vi "Open sequence.vi"(7 "Sequence name":string, 11 "error in (no error)":errorcluster) -> (4 "User input 1":T1, 6 "string steps":string[](array[string]), 8 "Steps":T2[](array[typedef]), 10 "Problem reading sequence":bool, 15 "error out":errorcluster)   [LabVIEW 2011]
uses:
  Sequence steps config..ctl
  Single criteria cluster.ctl
  Criteria types.ctl
  Boolean operation.ctl
  User input.ctl
  <vilib>/Utility/config.llb/NI_LVConfig.lvlib
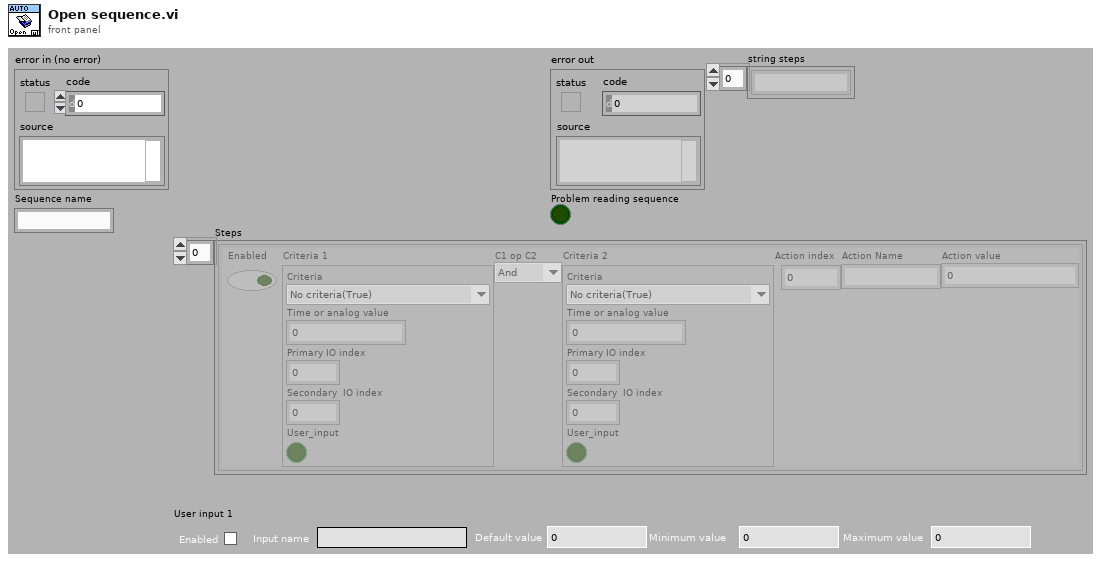
[diagram p1: front panel]
types:
  T1 = typedef "User input.ctl" = cluster{"Input name":string, "Minimum value ":dbl, "Maximum value":dbl, "Default value":dbl, "User inp enabled":bool}
  T2 = typedef "Sequence steps config..ctl" = cluster{"Enabled":bool, "Criteria 1":T3, "C1 op C2":T5, "Criteria 2":T3, "Action index":i32, "Action Name":string, "Action value":dbl}
  T3 = typedef "Single criteria cluster.ctl" = cluster{"Criteria":T4, "Time or analog value":dbl, "Primary IO index":i32, "Secondary  IO index":i32, "User_input":bool}
  T4 = typedef "Criteria types.ctl" = enum16{"No criteria(True)", "Time(s)", "Analog IO over", "Analog IO over or equal", "Analog IO under", "Analog IO under or equal", "Analog IO 1 minus Analog IO 2 over", "Digital IO True", "Digital IO False", "Operator approval"}
  T5 = typedef "Boolean operation.ctl" = enum16{"And", "Or", "Xor", "Nand", "Nor", "Nxor", "Implies"}
  T6 = typedef "NI_LVConfig.lvlib/Config Data RefNum.ctl" = refnum<k1>
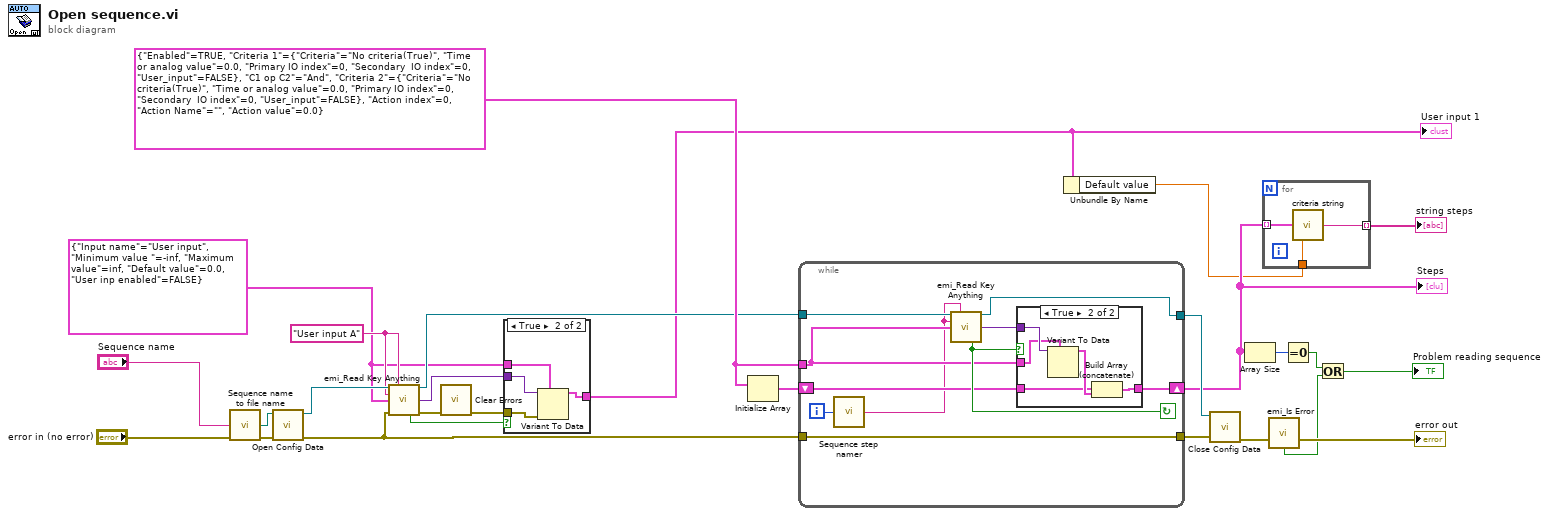
[diagram p0: block diagram]
diagram:
  w3 = T1 {"Input name"="User input", "Minimum value "=-inf, "Maximum value"=inf, "Default value"=0.0, "User inp enabled"=FALSE} ("User input 1")
  w7 = "User input A" ("Section(Default)")
  w21 = T2 {"Enabled"=TRUE, "Criteria 1"={"Criteria"=enum."No criteria(True)", "Time or analog value"=0.0, "Primary IO index"=0, "Secondary  IO index"=0, "User_input"=FALSE}, "C1 op C2"=enum."And", "Criteria 2"={"Criteria"=enum."No criteria(True)", "Time or analog value"=0.0, "Primary IO index"=0, "Secondary  IO index"=0, "User_input"=FALSE}, "Action index"=0, "Action Name"="", "Action value"=0.0} ("data step cluster")
  n1 = call "Sequence name to file name.vi"("Sequence name"="Sequence name", "error in (no error)"="error in (no error)") -> ("Sequence file path"=w25:path, "error out"=w24:errorcluster)  [unwired: 12 in]
  n2 = call <vilib>:"Open Config Data.vi"("error in (no error)"=w24, "configuration file path"=w25) -> ("error out"=w11:errorcluster, "refnum"=w9:T6)  [unwired: 7 in, 1 out]
  n3 = call "emi_Read Key Anything.vi"("Ini file refnum"=w9, "Section(Default)"=w7, "Name"=w7, "Anything"=w3, "error in (no error)"=w11) -> ("Ini file refnum out"=w8:T6, "Anything Out"=w6:variant, "Found"=w5:bool, "error out"=w10:errorcluster)  [unwired: 7 in]
  n4 = call <vilib>:"Clear Errors.vi"("error in (no error)"=w10) -> ("error out"=w4:errorcluster)  [unwired: 6 in]
  n5 = case shown="True" w5 {
    tunnel: w6 -> [_ w32]
    tunnel: w3 -> [w28 w31]
    tunnel: w4 -> [_ w30]
    tunnel: [w28 w29] -> w2
    frame False {
    }
    frame True {
      n6 = Variant To Data(error in=w30, type=w31, Variant=w32) -> (data=w29:T1)  [unwired: 1 out]
    }
  }
  "User input 1" <- w2
  n7 = Initialize Array(w21) -> (w20:T2[])  [unwired: 1 in]
  n8 = while {
    tunnel: w8 -> [w37]
    tunnel: w21 -> [w38]
    shift-right: [w41] -> w13
    shift-left: w20 -> [w40]
    tunnel: [w33] -> w22
    tunnel: w11 -> [w35]
    tunnel: [w35] -> w23
    i -> [w36]
    stop <- w42 continue-if-true
    n9 = call "Sequence step namer.vi"("number"=w36) -> ("Step name"=w34:string)
    n10 = call "emi_Read Key Anything.vi"("Ini file refnum"=w37, "Section(Default)"=w34, "Name"=w34, "Anything"=w38) -> ("Ini file refnum out"=w33:T6, "Anything Out"=w39:variant, "Found"=w42:bool)  [unwired: 8 in, 1 out]
    n11 = case shown="True" w42 {
      tunnel: [w43 w45] -> w41
      tunnel: w40 -> [w43 w44]
      tunnel: w39 -> [_ w48]
      tunnel: w38 -> [_ w47]
      frame False {
      }
      frame True {
        n12 = Variant To Data(type=w47, Variant=w48) -> (data=w46:T2)  [unwired: 1 in, 1 out]
        n13 = Build Array (concatenate)(w44, w46) -> (w45:T2[])
      }
    }
  }
  "Steps" <- w13
  n14 = Unbundle By Name(w2) -> ("Default value"=w1:dbl)
  n15 = call <vilib>:"Close Config Data.vi"("error in (no error)"=w23, "refnum"=w22) -> ("error out"=w19:errorcluster)  [unwired: 8 in, 1 out]
  n16 = Array Size(array=w13) -> (size(s)=w17:i32)
  n17 = for {
    tunnel: w13 -> [w51] mode=indexing
    tunnel: [w50] -> w12 mode=indexing
    tunnel: w1 -> [w49]
    n18 = call "criteria string.vi"("Sequence step config"=w51, "User input"=w49) -> ("Full criteria string"=w50:string)  [unwired: 12 in, 1 out]
  }
  "string steps" <- w12
  n19 = call "emi_Is Error.vi"("error in (no error)"=w19) -> ("error out"=→"error out":errorcluster, "Is Error"=w15:bool)  [unwired: 13 in]
  n20 = Equal To 0?(x=w17) -> (x = 0?=w16:bool)
  n21 = Or(x=w16, y=w15) -> (x .or. y?=→"Problem reading sequence":bool)
